vi "TWO AXIS (Incremental Input), automated.vi"() -> ()   [LabVIEW 2014]
uses:
  Control 1.ctl
  <vilib>/Instr/_visa.llb/VISA Flush IO Buffer Mask.ctl
  <vilib>/Instr/_visa.llb/VISA Configure Serial Port (Instr).vi
panel:
  in  "Mechanical X max":dbl
  in  "Mechanical Y max":dbl
  in  "X Min":dbl
  in  "Y Increment":dbl
  in  "Y Max":dbl
  in  "Y Min":dbl
  in  "X Increment":dbl
  in  "X Max":dbl
  in  "?":bool
  # "All Values are in cm."
  # "System operates by moving to a given Y-Value,\nthen iterates through all X values. After all Y-Values\nare complete the program waits for user confirmation\nthen returns to (0,0)."
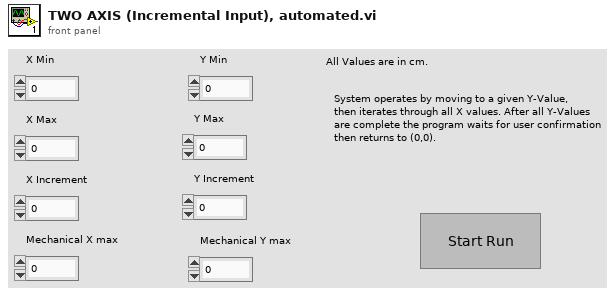
[diagram p1: front panel]
types:
  T1 = typedef "Control 1.ctl" = enum16{"Start", "Init", "Await Arduino Response", "Calculate Move", "Execute Move", "Home"}
  T2 = typedef "VISA Flush IO Buffer Mask.ctl" = u16
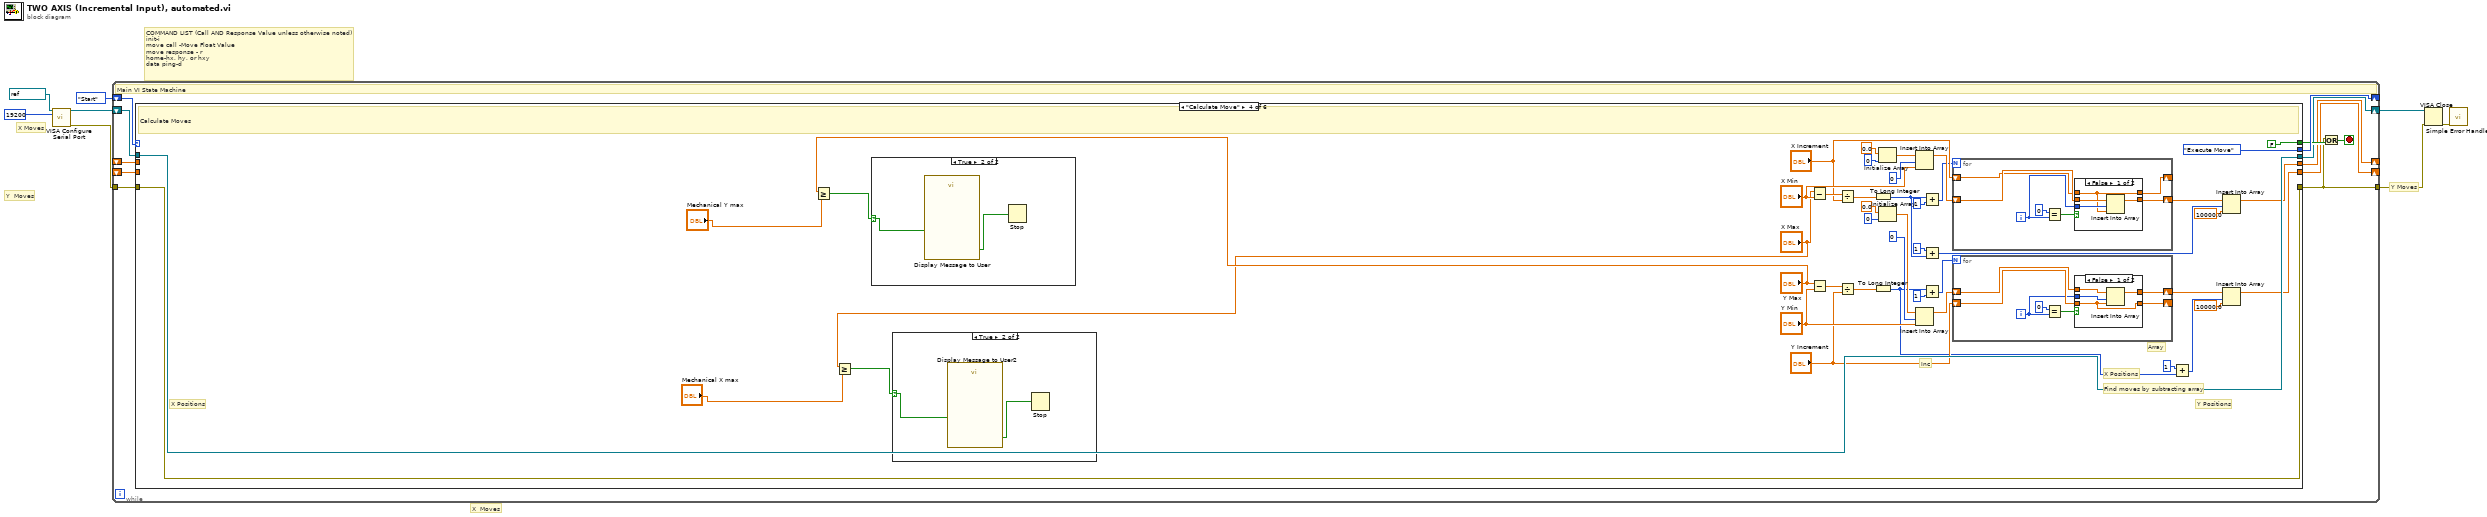
[diagram p0: block diagram]
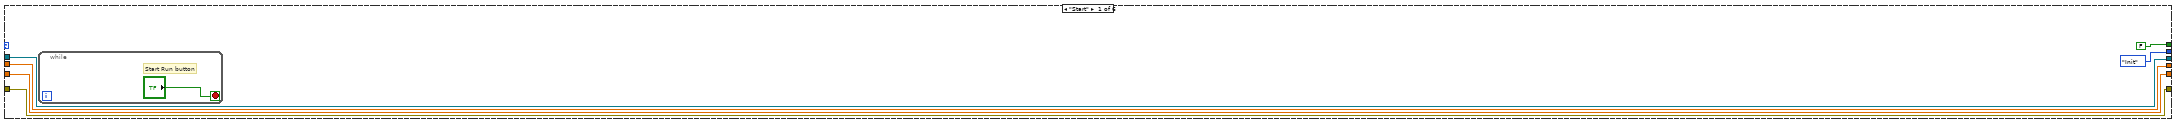
[diagram p2: hidden frame]
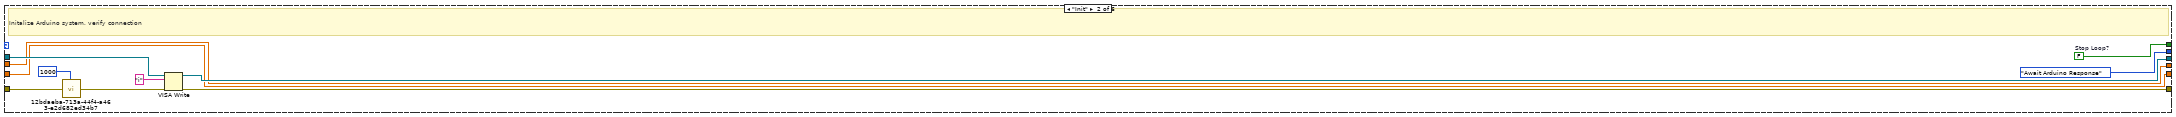
[diagram p3: hidden frame]
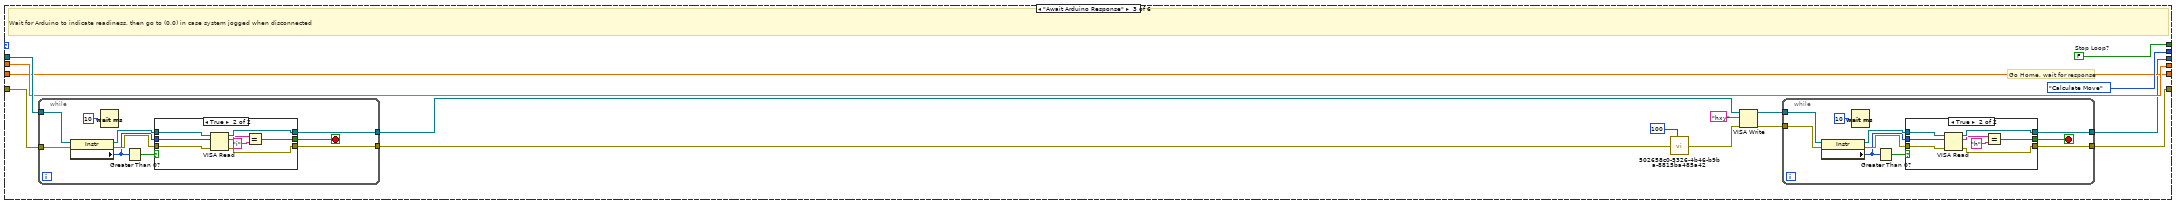
[diagram p4: hidden frame]
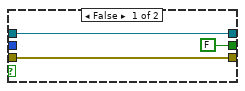
[diagram p5: hidden frame]
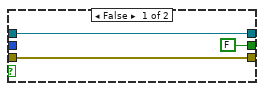
[diagram p6: hidden frame]
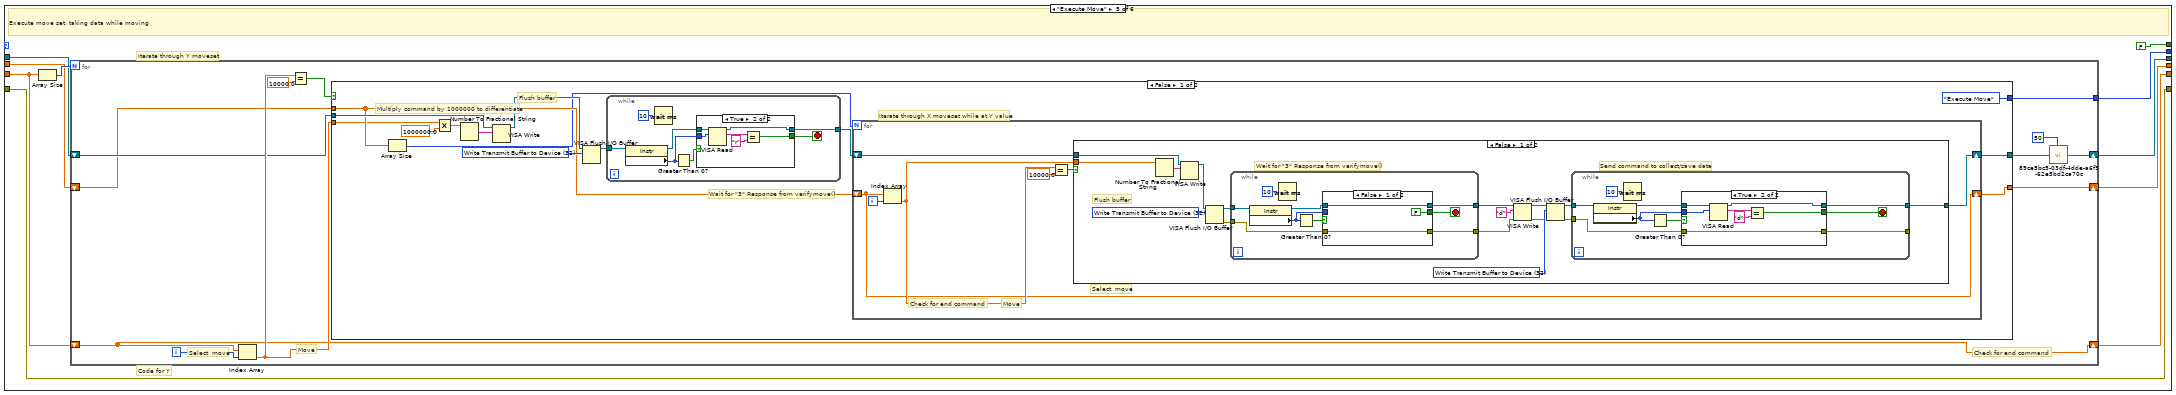
[diagram p11: hidden frame]
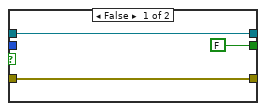
[diagram p12: hidden frame]
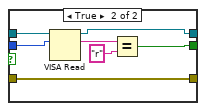
[diagram p13: hidden frame]
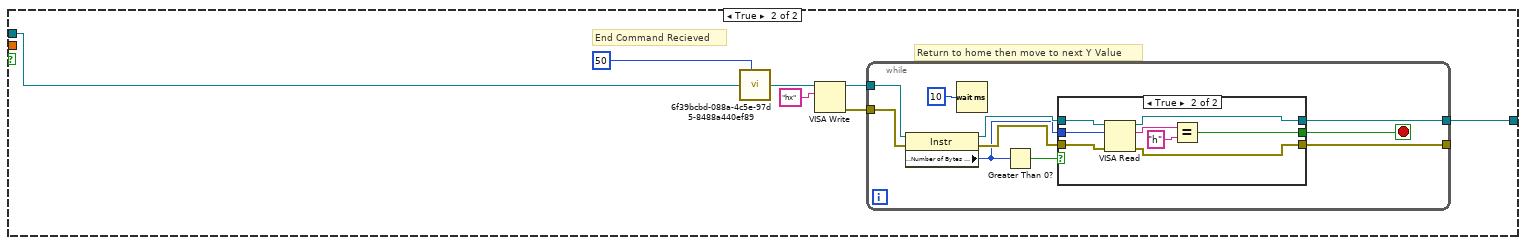
[diagram p14: hidden frame]
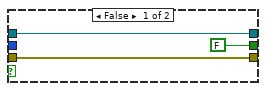
[diagram p15: hidden frame]
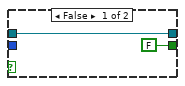
[diagram p16: hidden frame]
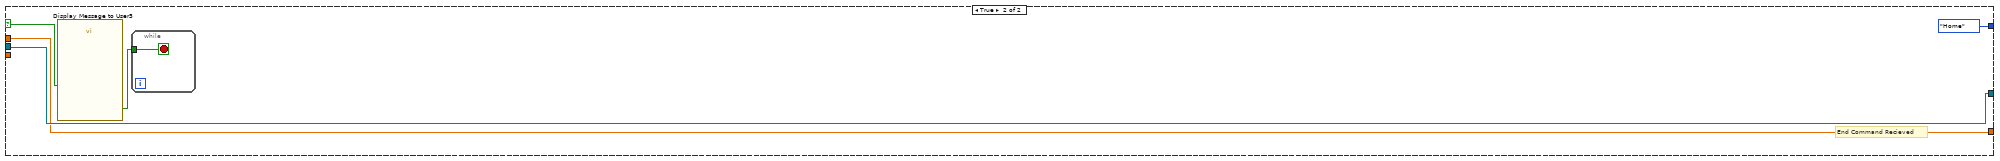
[diagram p17: hidden frame]
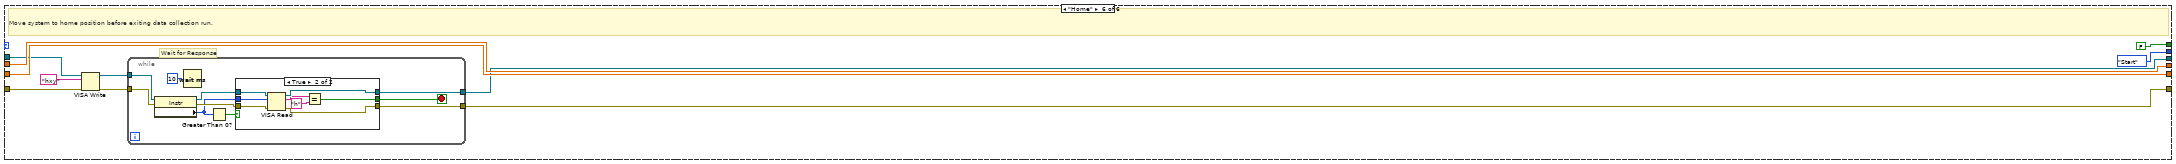
[diagram p18: hidden frame]
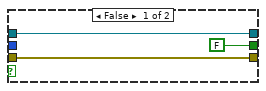
[diagram p19: hidden frame]
diagram:
  # "X  Moves"
  # "COMMAND LIST (Call AND Response Value unless otherwise noted)\ninit-i\nmove call -Move Float Value\nmove response - r\nhome-hx, hy, or hxy\ndata ping-d"
  # "Y Moves"
  # "X Moves"
  # "Y  Moves"
  n1 = call-poly "VISA Configure Serial Port"("VISA resource name"=refnum<visa-resource-name> "COM9", "baud rate (9600)"=u32 19200) -> ("VISA resource name out"=w6:refnum<visa-resource-name>, "error out"=w2:errorcluster)  [unwired: 12 in]
  n2 = while {
    shift-right: [w19] -> _
    shift-left: Control_1."Start" -> [w20]
    shift-right: [w16] -> w5
    shift-left: w6 -> [w17]
    shift-right: [w15] -> _
    shift-left: _ -> [w13]
    shift-right: [w14] -> _
    shift-left: _ -> [w12]
    tunnel: w2 -> [w11]
    tunnel: [w10] -> w1
    stop <- w9 stop-if-true
    # "Main VI State Machine"
    n3 = case shown="\"Calculate Move\"" w20 {
      tunnel: [Control_1."Init" Control_1."Await Arduino Response" Control_1."Calculate Move" Control_1."Execute Move" w173 Control_1."Start"] -> w19
      tunnel: [FALSE ("Stop Loop?") w38 w53 FALSE FALSE FALSE ("Stop Loop?")] -> w18
      tunnel: w17 -> [w23 w32 w52 w137 w170 w322]
      tunnel: w11 -> [w24 w34 w51 w136 w174 w321]
      tunnel: [w23 w35 w40 w137 w175 w317] -> w16
      tunnel: [w24 w36 w39 w136 w174 w316] -> w10
      tunnel: [w26 w29 w49 w103 w171 w324] -> w15
      tunnel: [w25 w28 w48 w102 w176 w323] -> w14
      tunnel: w13 -> [w26 w29 w49 _ w172 w324]
      tunnel: w12 -> [w25 w28 w48 _ w177 w323]
      frame "Start" {
        n4 = while {
          stop <- "?" stop-if-true
          # "Start Run button"
        }
      }
      frame "Init" {
        w38 = FALSE  # Stop Loop?
        # "Initalize Arduino system, verify connection"
        n5 = call "12bdaeba-713a-44f4-a463-e2d682ed34b7.vi"("value in"=w34, "milliseconds to wait"=u32 1000) -> ("value out"=w33:errorcluster)  [unwired: 1 out]
        n6 = VISA Write(VISA resource name=w32, write buffer="i", error in (no error)=w33) -> (VISA resource name out=w35:refnum<visa-resource-name>, error out=w36:errorcluster)  [unwired: 1 out]
      }
      frame "Await Arduino Response" {
        w53 = FALSE  # Stop Loop?
        # "Go Home, wait for response"
        # "Wait for Arduino to indicate readiness, then go to (0,0) in case system jogged when disconnected"
        n7 = while {
          tunnel: w52 -> [w84]
          tunnel: w51 -> [w83]
          tunnel: [w77] -> w42
          tunnel: [w76] -> w47
          stop <- w78 stop-if-true
          n8 = property class="Instr"(reference=w84, error in=w83) -> (reference out=w81:refnum<visa-resource-name>, error out=w80:errorcluster, "Serial Settings:Number of Bytes at Serial Port"=w79:u32)
          n9 = Wait (ms)(milliseconds to wait=u32 10) -> ()  [unwired: 1 out]
          n10 = Greater Than 0?(x=w79) -> (x > 0?=w82:bool)
          n11 = case shown="True" w82 {
            tunnel: w81 -> [w87 w95]
            tunnel: w80 -> [w86 w94]
            tunnel: w79 -> [_ w93]
            tunnel: [FALSE w89] -> w78
            tunnel: [w87 w91] -> w77
            tunnel: [w86 w90] -> w76
            frame False {
            }
            frame True {
              n12 = VISA Read(VISA resource name=w95, byte count=w93, error in (no error)=w94) -> (VISA resource name out=w91:refnum<visa-resource-name>, read buffer=w88:string, error out=w90:errorcluster)  [unwired: 1 out]
              n13 = Equal?(x=w88, y="i") -> (x = y?=w89:bool)
            }
          }
        }
        n14 = call "502658c0-5326-4b46-b9ba-8815ba485a42.vi"("value in"=w47, "milliseconds to wait"=u32 100) -> ("value out"=w41:errorcluster)  [unwired: 1 out]
        n15 = VISA Write(VISA resource name=w42, write buffer="hxy", error in (no error)=w41) -> (VISA resource name out=w44:refnum<visa-resource-name>, error out=w43:errorcluster)  [unwired: 1 out]
        n16 = while {
          tunnel: w44 -> [w63]
          tunnel: w43 -> [w62]
          tunnel: [w56] -> w40
          tunnel: [w55] -> w39
          stop <- w57 stop-if-true
          n17 = property class="Instr"(reference=w63, error in=w62) -> (reference out=w60:refnum<visa-resource-name>, error out=w59:errorcluster, "Serial Settings:Number of Bytes at Serial Port"=w58:u32)
          n18 = Wait (ms)(milliseconds to wait=u32 10) -> ()  [unwired: 1 out]
          n19 = Greater Than 0?(x=w58) -> (x > 0?=w61:bool)
          n20 = case shown="True" w61 {
            tunnel: w60 -> [w66 w74]
            tunnel: w59 -> [w65 w73]
            tunnel: w58 -> [_ w72]
            tunnel: [FALSE w68] -> w57
            tunnel: [w66 w70] -> w56
            tunnel: [w65 w69] -> w55
            frame False {
            }
            frame True {
              n21 = VISA Read(VISA resource name=w74, byte count=w72, error in (no error)=w73) -> (VISA resource name out=w70:refnum<visa-resource-name>, read buffer=w67:string, error out=w69:errorcluster)  [unwired: 1 out]
              n22 = Equal?(x=w67, y="h") -> (x = y?=w68:bool)
            }
          }
        }
      }
      frame "Calculate Move" {
        # "Inc"
        # "Array"
        # "X Positions"
        # "Find moves by subtracting array"
        # "X Positions"
        # "Y Positions"
        # "Calculate Moves"
        n23 = Greater Or Equal?(x="Y Max", y="Mechanical Y max") -> (x >= y?=w101:bool)
        n24 = Greater Or Equal?(x="X Max", y="Mechanical X max") -> (x >= y?=w100:bool)
        n25 = case shown="True" w101 {
          selector: w101 -> [_ w143]
          frame False {
          }
          frame True {
            n26 = call "Display Message to User"("Enable"=w143) -> ("OK"=w142:bool)  [unwired: 9 in, 1 out]
            n27 = Stop(stop? (T)=w142) -> ()
          }
        }
        n28 = case shown="True" w100 {
          selector: w100 -> [_ w140]
          frame False {
          }
          frame True {
            n29 = call "Display Message to User2"("Enable"=w140) -> ("OK"=w141:bool)  [unwired: 9 in, 1 out]
            n30 = Stop(stop? (T)=w141) -> ()
          }
        }
        n31 = Subtract(x="X Max", y="X Min") -> (x-y=w134:dbl)
        n32 = Subtract(x="Y Max", y="Y Min") -> (x-y=w135:dbl)
        n33 = Divide(x=w134, y="X Increment") -> (x/y=w133:dbl)
        n34 = Divide(x=w135, y="Y Increment") -> (x/y=w132:dbl)
        n35 = To Long Integer(number=w133) -> (32bit integer=w107:i32)
        n36 = To Long Integer(number=w132) -> (32bit integer=w111:i32)
        n37 = Initialize Array(0.0 ("element"), 0 ("dimension size")) -> (w120:dbl[])
        n38 = Initialize Array(0.0 ("element"), 0 ("dimension size")) -> (w123:dbl[])
        n39 = Insert Into Array(array=w120, index=0, new element="X Min") -> (w116:dbl[])
        n40 = Insert Into Array(array=w123, index=0, new element="Y Min") -> (w119:dbl[])
        n41 = Add(x=w107, y=1) -> (x+y=w114:i32)
        n42 = Add(x=1, y=w107) -> (x+y=w105:i32)
        n43 = Add(x=w111, y=1) -> (x+y=w117:i32)
        n44 = for {
          N: w114 -> [_]
          shift-right: [w147] -> w108
          shift-left: w116 -> [w148]
          shift-right: [w145] -> _
          shift-left: "X Increment" -> [w146]
          i -> [w144]
          n45 = Equal?(x=0, y=w144) -> (x = y?=w149:bool)
          n46 = case shown="False" w149 {
            tunnel: w148 -> [w153 w156]
            tunnel: [w152 w156] -> w147
            tunnel: w146 -> [w151 w155]
            tunnel: [w151 w155] -> w145
            tunnel: w144 -> [w154 _]
            frame False {
              n47 = Insert Into Array(array=w153, index=w154, new element=w151) -> (w152:dbl[])
            }
            frame True {
            }
          }
        }
        n48 = for {
          N: w117 -> [_]
          shift-right: [w160] -> w113
          shift-left: w119 -> [w161]
          shift-right: [w158] -> _
          shift-left: "Y Increment" -> [w159]
          i -> [w157]
          n49 = Equal?(x=0, y=w157) -> (x = y?=w162:bool)
          n50 = case shown="False" w162 {
            tunnel: w161 -> [w166 w169]
            tunnel: [w165 w169] -> w160
            tunnel: w159 -> [w164 w168]
            tunnel: [w164 w168] -> w158
            tunnel: w157 -> [w167 _]
            frame False {
              n51 = Insert Into Array(array=w166, index=w167, new element=w164) -> (w165:dbl[])
            }
            frame True {
            }
          }
        }
        n52 = Add(x=1, y=w111) -> (x+y=w109:i32)
        n53 = Insert Into Array(array=w108, index=w105, new element=10000.0 ("new element/subarray")) -> (w103:dbl[])
        n54 = Insert Into Array(array=w113, index=w109, new element=10000.0 ("new element/subarray")) -> (w102:dbl[])
      }
      frame "Execute Move" {
        # "Iterate through Y moveset"
        # "Code for Y"
        # "Execute move set, taking data while moving"
        n55 = Array Size(array=w177) -> (size(s)=w178:i32)
        n56 = for {
          N: w178 -> [_]
          shift-right: [w187] -> w176
          shift-left: w177 -> [w187]
          tunnel: [w186] -> w173
          shift-right: [w183] -> w175
          shift-left: w170 -> [w185]
          shift-right: [w180] -> w171
          shift-left: w172 -> [w181]
          i -> [w191]
          # "Select  move"
          # "Check for end command"
          # "Move"
          n57 = Index Array(array=w187, index=w191) -> (element=w188:dbl)
          n58 = Equal?(x=w188, y=10000.0) -> (x = y?=w189:bool)
          n59 = case shown="False" w189 {
            selector: w189 -> [_ w313]
            tunnel: w188 -> [w194 _]
            tunnel: [Control_1."Execute Move" Control_1."Home"] -> w186
            tunnel: w185 -> [w204 w311]
            tunnel: [w197 w311] -> w184
            tunnel: w181 -> [w196 w310]
            tunnel: [w198 w310] -> w180
            frame False {
              w200 = T2 32 items=["Flush Receive Buffer"=16, "Write Transmit Buffer to Device"=32, "Flush Receive Buffer (No I/O)"=64, "Flush Transmit Buffer"=128] ("Mask")
              # "Flush buffer"
              # "Iterate through X moveset while at Y value"
              # "Multiply command by 1000000 to differentiate"
              # "Wait for \"3\" Response from verifymove()"
              n60 = Array Size(array=w196) -> (size(s)=w195:i32)
              n61 = Multiply(x=w194, y=1000000.0) -> (x*y=w193:dbl)
              n62 = Number To Fractional String(number=w193) -> (F-format string=w203:string)  [unwired: 3 in]
              n63 = VISA Write(VISA resource name=w204, write buffer=w203) -> (VISA resource name out=w202:refnum<visa-resource-name>)  [unwired: 1 in, 2 out]
              n64 = VISA Flush I/O Buffer(VISA resource name=w202, mask (16)=w200) -> (VISA resource name out=w201:refnum<visa-resource-name>)  [unwired: 1 in, 1 out]
              n65 = while {
                tunnel: w201 -> [w301]
                tunnel: [w296] -> w199
                stop <- w297 stop-if-true
                n66 = property class="Instr"(reference=w301) -> (reference out=w299:refnum<visa-resource-name>, "Serial Settings:Number of Bytes at Serial Port"=w298:u32)  [unwired: 1 in, 1 out]
                n67 = Wait (ms)(milliseconds to wait=u32 10) -> ()  [unwired: 1 out]
                n68 = Greater Than 0?(x=w298) -> (x > 0?=w300:bool)
                n69 = case shown="True" w300 {
                  tunnel: w299 -> [w303 w309]
                  tunnel: w298 -> [_ w308]
                  tunnel: [FALSE w306] -> w297
                  tunnel: [w303 w307] -> w296
                  frame False {
                  }
                  frame True {
                    n70 = VISA Read(VISA resource name=w309, byte count=w308) -> (VISA resource name out=w307:refnum<visa-resource-name>, read buffer=w305:string)  [unwired: 1 in, 2 out]
                    n71 = Equal?(x=w305, y="r") -> (x = y?=w306:bool)
                  }
                }
              }
              n72 = for {
                N: w195 -> [_]
                shift-right: [w207] -> w198
                shift-left: w196 -> [w207]
                shift-right: [w206] -> w197
                shift-left: w199 -> [w208]
                i -> [w212]
                # "Check for end command"
                # "Move"
                # "Select  move"
                n73 = Index Array(array=w207, index=w212) -> (element=w209:dbl)
                n74 = Equal?(x=w209, y=10000.0) -> (x = y?=w210:bool)
                n75 = case shown="False" w210 {
                  tunnel: w209 -> [w227 _]
                  tunnel: w208 -> [w228 w269]
                  tunnel: [w215 w270] -> w206
                  frame False {
                    w216 = T2 32 items=["Flush Receive Buffer"=16, "Write Transmit Buffer to Device"=32, "Flush Receive Buffer (No I/O)"=64, "Flush Transmit Buffer"=128] ("Mask")
                    w223 = T2 32 items=["Flush Receive Buffer"=16, "Write Transmit Buffer to Device"=32, "Flush Receive Buffer (No I/O)"=64, "Flush Transmit Buffer"=128] ("Mask")
                    # "Send command to collect/save data"
                    # "Flush buffer"
                    # "Wait for \"3\" Response from verifymove()"
                    n76 = Number To Fractional String(number=w227) -> (F-format string=w226:string)  [unwired: 3 in]
                    n77 = VISA Write(VISA resource name=w228, write buffer=w226) -> (VISA resource name out=w225:refnum<visa-resource-name>)  [unwired: 1 in, 2 out]
                    n78 = VISA Flush I/O Buffer(VISA resource name=w225, mask (16)=w223) -> (VISA resource name out=w224:refnum<visa-resource-name>, error out=w222:errorcluster)  [unwired: 1 in]
                    n79 = while {
                      tunnel: w224 -> [w256]
                      tunnel: [w251] -> w218
                      tunnel: w222 -> [w249]
                      tunnel: [w248] -> w214
                      stop <- w252 stop-if-true
                      n80 = property class="Instr"(reference=w256) -> (reference out=w254:refnum<visa-resource-name>, "Serial Settings:Number of Bytes at Serial Port"=w253:u32)  [unwired: 1 in, 1 out]
                      n81 = Wait (ms)(milliseconds to wait=u32 10) -> ()  [unwired: 1 out]
                      n82 = Greater Than 0?(x=w253) -> (x > 0?=w255:bool)
                      n83 = case shown="False" w255 {
                        tunnel: w254 -> [w259 w266]
                        tunnel: w253 -> [_ w265]
                        tunnel: [FALSE w263] -> w252
                        tunnel: [w259 w264] -> w251
                        tunnel: w249 -> [w257 w260]
                        tunnel: [w257 w260] -> w248
                        frame False {
                        }
                        frame True {
                          n84 = VISA Read(VISA resource name=w266, byte count=w265) -> (VISA resource name out=w264:refnum<visa-resource-name>, read buffer=w262:string)  [unwired: 1 in, 2 out]
                          n85 = Equal?(x=w262, y="r") -> (x = y?=w263:bool)
                        }
                      }
                    }
                    n86 = VISA Write(VISA resource name=w218, write buffer="d", error in (no error)=w214) -> (VISA resource name out=w221:refnum<visa-resource-name>, error out=w213:errorcluster)  [unwired: 1 out]
                    n87 = VISA Flush I/O Buffer(VISA resource name=w221, mask (16)=w216, error in (no error)=w213) -> (VISA resource name out=w220:refnum<visa-resource-name>, error out=w219:errorcluster)
                    n88 = while {
                      tunnel: w220 -> [w237]
                      tunnel: [w232] -> w215
                      tunnel: w219 -> [w230]
                      tunnel: [w229] -> _
                      stop <- w233 stop-if-true
                      n89 = property class="Instr"(reference=w237) -> (reference out=w235:refnum<visa-resource-name>, "Serial Settings:Number of Bytes at Serial Port"=w234:u32)  [unwired: 1 in, 1 out]
                      n90 = Wait (ms)(milliseconds to wait=u32 10) -> ()  [unwired: 1 out]
                      n91 = Greater Than 0?(x=w234) -> (x > 0?=w236:bool)
                      n92 = case shown="True" w236 {
                        tunnel: w235 -> [w240 w247]
                        tunnel: w234 -> [_ w246]
                        tunnel: [FALSE w244] -> w233
                        tunnel: [w240 w245] -> w232
                        tunnel: w230 -> [w238 w241]
                        tunnel: [w238 w241] -> w229
                        frame False {
                        }
                        frame True {
                          n93 = VISA Read(VISA resource name=w247, byte count=w246) -> (VISA resource name out=w245:refnum<visa-resource-name>, read buffer=w243:string)  [unwired: 1 in, 2 out]
                          n94 = Equal?(x=w243, y="d") -> (x = y?=w244:bool)
                        }
                      }
                    }
                  }
                  frame True {
                    # "Return to home then move to next Y Value"
                    # "End Command Recieved"
                    n95 = call "6f39bcbd-088a-4c5e-97d5-8488a440ef89.vi"("value in"=w269, "milliseconds to wait"=u32 50) -> ("value out"=w268:refnum<visa-resource-name>)  [unwired: 1 out]
                    n96 = VISA Write(VISA resource name=w268, write buffer="hx") -> (VISA resource name out=w272:refnum<visa-resource-name>, error out=w271:errorcluster)  [unwired: 1 in, 1 out]
                    n97 = while {
                      tunnel: w272 -> [w283]
                      tunnel: w271 -> [w282]
                      tunnel: [w276] -> w270
                      tunnel: [w275] -> _
                      stop <- w277 stop-if-true
                      n98 = property class="Instr"(reference=w283, error in=w282) -> (reference out=w280:refnum<visa-resource-name>, error out=w279:errorcluster, "Serial Settings:Number of Bytes at Serial Port"=w278:u32)
                      n99 = Wait (ms)(milliseconds to wait=u32 10) -> ()  [unwired: 1 out]
                      n100 = Greater Than 0?(x=w278) -> (x > 0?=w281:bool)
                      n101 = case shown="True" w281 {
                        tunnel: w280 -> [w286 w294]
                        tunnel: w279 -> [w285 w293]
                        tunnel: w278 -> [_ w292]
                        tunnel: [FALSE w288] -> w277
                        tunnel: [w286 w290] -> w276
                        tunnel: [w285 w289] -> w275
                        frame False {
                        }
                        frame True {
                          n102 = VISA Read(VISA resource name=w294, byte count=w292, error in (no error)=w293) -> (VISA resource name out=w290:refnum<visa-resource-name>, read buffer=w287:string, error out=w289:errorcluster)  [unwired: 1 out]
                          n103 = Equal?(x=w287, y="h") -> (x = y?=w288:bool)
                        }
                      }
                    }
                  }
                }
              }
            }
            frame True {
              # "End Command Recieved"
              n104 = call "Display Message to User3"("Enable"=w313) -> ("Return to Home"=w314:bool)  [unwired: 9 in, 1 out]
              n105 = while {
                tunnel: w314 -> [w315]
                stop <- w315 stop-if-true
              }
            }
          }
          n106 = call "89ce5bc5-03df-4dde-a6f9-62e5bd2ca70c.vi"("value in"=w184, "milliseconds to wait"=u32 50) -> ("value out"=w183:refnum<visa-resource-name>)  [unwired: 1 out]
        }
      }
      frame "Home" {
        # "Wait for Response"
        # "Move system to home position before exiting data collection run."
        n107 = VISA Write(VISA resource name=w322, write buffer="hxy", error in (no error)=w321) -> (VISA resource name out=w319:refnum<visa-resource-name>, error out=w318:errorcluster)  [unwired: 1 out]
        n108 = while {
          tunnel: w319 -> [w336]
          tunnel: w318 -> [w335]
          tunnel: [w329] -> w317
          tunnel: [w328] -> w316
          stop <- w330 stop-if-true
          n109 = property class="Instr"(reference=w336, error in=w335) -> (reference out=w333:refnum<visa-resource-name>, error out=w332:errorcluster, "Serial Settings:Number of Bytes at Serial Port"=w331:u32)
          n110 = Wait (ms)(milliseconds to wait=u32 10) -> ()  [unwired: 1 out]
          n111 = Greater Than 0?(x=w331) -> (x > 0?=w334:bool)
          n112 = case shown="True" w334 {
            tunnel: w333 -> [w339 w347]
            tunnel: w332 -> [w338 w346]
            tunnel: w331 -> [_ w345]
            tunnel: [FALSE w341] -> w330
            tunnel: [w339 w343] -> w329
            tunnel: [w338 w342] -> w328
            frame False {
            }
            frame True {
              n113 = VISA Read(VISA resource name=w347, byte count=w345, error in (no error)=w346) -> (VISA resource name out=w343:refnum<visa-resource-name>, read buffer=w340:string, error out=w342:errorcluster)  [unwired: 1 out]
              n114 = Equal?(x=w340, y="h") -> (x = y?=w341:bool)
            }
          }
        }
      }
    }
    n115 = Or(x=w10, y=w18) -> (x .or. y?=w9:bool)
  }
  n116 = VISA Close(VISA resource name=w5, error in (no error)=w1) -> (error out=w7:errorcluster)
  n117 = call <vilib>:"Simple Error Handler.vi"("error in (no error)"=w7) -> ()  [unwired: 4 in, 5 out]
